vi "LHF.DB.Mongo.Collection.CreateIndex.vi"(8 "error in (no error)":errorcluster, 9 "value":variant, 10 "Collection":string, 11 "LHF.DB.Mongo in":refnum<class "LHF.DB.Mongo.lvclass">) -> (0 "error out":errorcluster, 1 "Ok":bool, 3 "LHF.DB.Mongo out":refnum<class "LHF.DB.Mongo.lvclass">)   [LabVIEW 2013, in "LHF.DB.Mongo.lvclass"]
doc: "Creates an index in collection. Variable name, type & content will be used."
uses:
  LHF.DB.Mongo.lvclass
  C:/Users/Ricardo/Desktop/Projetos/LabVIEW-MongoDB/src/Driver/MongoDB.Driver.dll
  Driver/MongoDB.Driver.dll
  <vilib>/Utility/VariantDataType/VariantType.lvlib
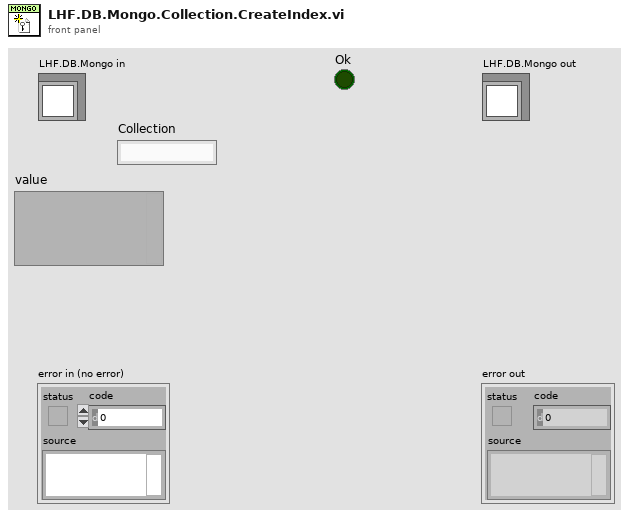
[diagram p1: front panel]
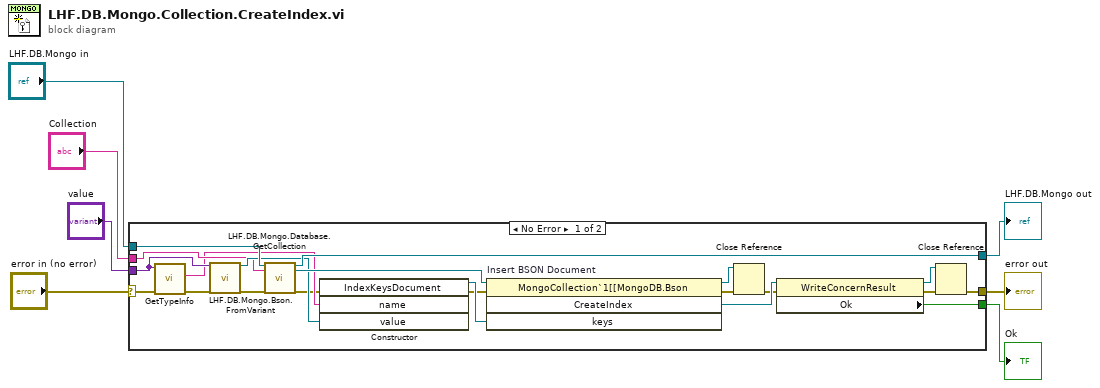
[diagram p0: block diagram]
diagram:
  n1 = case shown="No Error" "error in (no error)" {
    selector: "error in (no error)" -> [w16 w30]
    tunnel: [w8 w30] -> w6
    tunnel: [w26 w29] -> w4
    tunnel: "LHF.DB.Mongo in" -> [w27 w29]
    tunnel: "value" -> [w19 _]
    tunnel: "Collection" -> [w21 _]
    tunnel: [w11 _] -> w1
    frame No Error {
      n2 = call <vilib>:"GetTypeInfo.vi"("error in (no error)"=w16, "Variant"=w19) -> ("error out"=w17:errorcluster, "Name"=w18:string)  [unwired: 5 in, 3 out]
      n3 = call "LHF.DB.Mongo.Bson.FromVariant.vi"("Variant"=w19, "error IO"=w17) -> ("BsonValue"=w24:refnum<k24>, "error IO 2"=w15:errorcluster)  [unwired: 16 in]
      n4 = call "LHF.DB.Mongo.Database.GetCollection.vi"("LHF.DB.Mongo in"=w27, "collectionName"=w21, "error in (no error)"=w15) -> ("LHF.DB.Mongo in"=w26:refnum<class "LHF.DB.Mongo.lvclass">, "MongoCollection"=w25:refnum<k24>, "error out"=w14:errorcluster)  [unwired: 14 in]
      n5 = constructor class="IndexKeysDocument"(error in=w14, "name"=w18, "value"=w24) -> (reference out=w28:refnum<k24>, error out=w23:errorcluster)  [unwired: 2 in, 3 out]
      n6 = invoke on="Insert BSON Document" class="MongoCollection`1[[MongoDB.Bson" method="CreateIndex"(reference=w25, error in=w23, "keys"=w28) -> (reference out=w20:refnum<k24>, error out=w22:errorcluster, "CreateIndex"=w13:refnum<k24>)  [unwired: 1 in, 1 out]
      n7 = Close Reference(reference=w20, error in (no error)=w22) -> (error out=w12:errorcluster)
      n8 = property class="WriteConcernResult"(reference=w13, error in=w12) -> (reference out=w10:refnum<k24>, error out=w9:errorcluster, "Ok"=w11:bool)
      n9 = Close Reference(reference=w10, error in (no error)=w9) -> (error out=w8:errorcluster)
    }
    frame Error {
    }
  }
  "error out" <- w6
  "LHF.DB.Mongo out" <- w4
  "Ok" <- w1
